vi "CompareXML.vi"(6 "Native LV Version":string, 7 "Lv Version":string, 8 "error in":errorcluster, 9 "file path (use dialog)":path=path "C:/Users/Localization Tester/Desktop/Reporting", 10 "name or relative path":string, 11 "Failure_DB__File_Paths_Array":path[](array[path])) -> (0 "error out":errorcluster, 3 "XML File Path(duplicate)":path)   [LabVIEW 2012]
uses:
  Data.ctl
  Write to XML File(string).vi
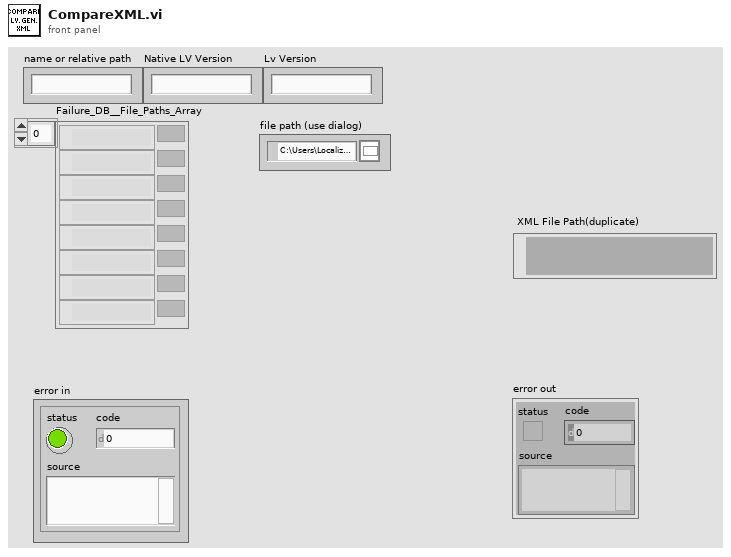
[diagram p1: front panel]
types:
  T1 = typedef "Data.ctl" = cluster{"VI":string[], "Status":enum16{"", "new", "passed", "known"}, "Crash":bool, "Linux":bool, "Mac":bool, "Windows":bool, "Comments":string, "First Reported":timestamp, "CAR":string, "Paused":bool, "failure_desc":cluster{"desc":string, "type":enum32{"generic failure", "boundary case", "precision", "expected error"}}[], "Id":i32}
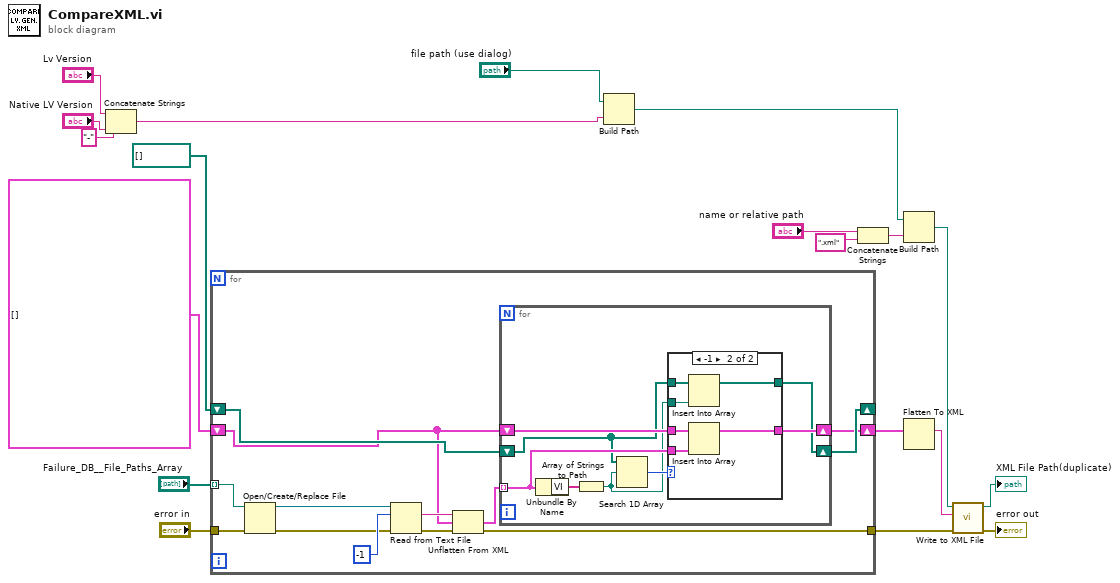
[diagram p0: block diagram]
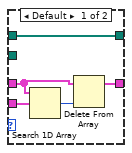
[diagram p2: hidden frame]
diagram:
  n1 = Concatenate Strings("Lv Version", "-" ("string"), "Native LV Version") -> (w4:string)
  n2 = for {
    tunnel: "Failure_DB__File_Paths_Array" -> [w26] mode=indexing
    shift-right: [w24] -> w15
    shift-left: T1[] [] ("Loaded Data in") -> [w25]
    shift-right: [w29] -> _
    shift-left: path[] [] -> [w28]
    tunnel: "error in" -> [w21]
    tunnel: [w20] -> w13
    n3 = Open/Create/Replace File(file path (use dialog)=w26, error in=w21) -> (refnum out=w30:refnum<file>, error out=w23:errorcluster)  [unwired: 4 in, 1 out]
    n4 = Read from Text File(file (use dialog)=w30, count=-1, error in=w23) -> (text=w32:string, error out=w22:errorcluster)  [unwired: 1 in, 2 out]
    n5 = Unflatten From XML(xml string=w32, type=w25, error in (no error)=w22) -> (value=w27:T1[], error out=w20:errorcluster)
    n6 = for {
      tunnel: w27 -> [w38] mode=indexing
      shift-right: [w34] -> w29
      shift-left: w28 -> [w35]
      shift-right: [w36] -> w24
      shift-left: w25 -> [w37]
      n7 = Unbundle By Name(w38) -> ("VI"=w40:string[])
      n8 = Array of Strings to Path(0:w40) -> (2:w33:path)  [unwired: 1 in]
      n9 = Search 1D Array(1D array=w35, element=w33) -> (index of element=w39:i32)  [unwired: 1 in]
      n10 = case shown="-1" w39 {
        tunnel: w38 -> [w42 w50]
        tunnel: w37 -> [w43 w51]
        tunnel: [w44 w49] -> w36
        tunnel: w35 -> [w45 w48]
        tunnel: [w45 w47] -> w34
        tunnel: w33 -> [_ w46]
        frame Default {
          n11 = Search 1D Array(1D array=w43, element=w42) -> (index of element=w41:i32)  [unwired: 1 in]
          n12 = Delete From Array(array=w43, index=w41) -> (array with subset deleted=w44:T1[])  [unwired: 1 in, 1 out]
        }
        frame -1 {
          n13 = Insert Into Array(array=w48, new element=w46) -> (w47:path[])  [unwired: 1 in]
          n14 = Insert Into Array(array=w51, new element=w50) -> (w49:T1[])  [unwired: 1 in]
        }
      }
    }
  }
  n15 = Build Path(base path="file path (use dialog)", name or relative path=w4) -> (appended path=w3:path)
  n16 = Concatenate Strings("name or relative path", ".xml" ("string")) -> (w9:string)
  n17 = Build Path(base path=w3, name or relative path=w9) -> (appended path=w1:path)
  n18 = Flatten To XML(anything=w15) -> (xml string=w2:string)
  n19 = call-poly <vilib>:"Write to XML File.vi"("error in (no error)"=w13, "XML Input"=w2, "XML File Path"=w1) -> ("error out"=→"error out":errorcluster, "XML File Path(duplicate)"=→"XML File Path(duplicate)":path)  [unwired: 6 in, 1 out]
